vi "_TBD Get Templates Folder Location.vi"() -> (0 "Templates Folder Location":path)   [LabVIEW 2022 SP3]
doc: "Returns the folder location where template VIs and/or CTLs are expected to be found."
panel:
  # "Development\ncontrols/indicators useful for development and testing, but which are not outputs of the VI"
  # "Input\nInputs to the VI"
  # "Output\nOutputs of the VI"
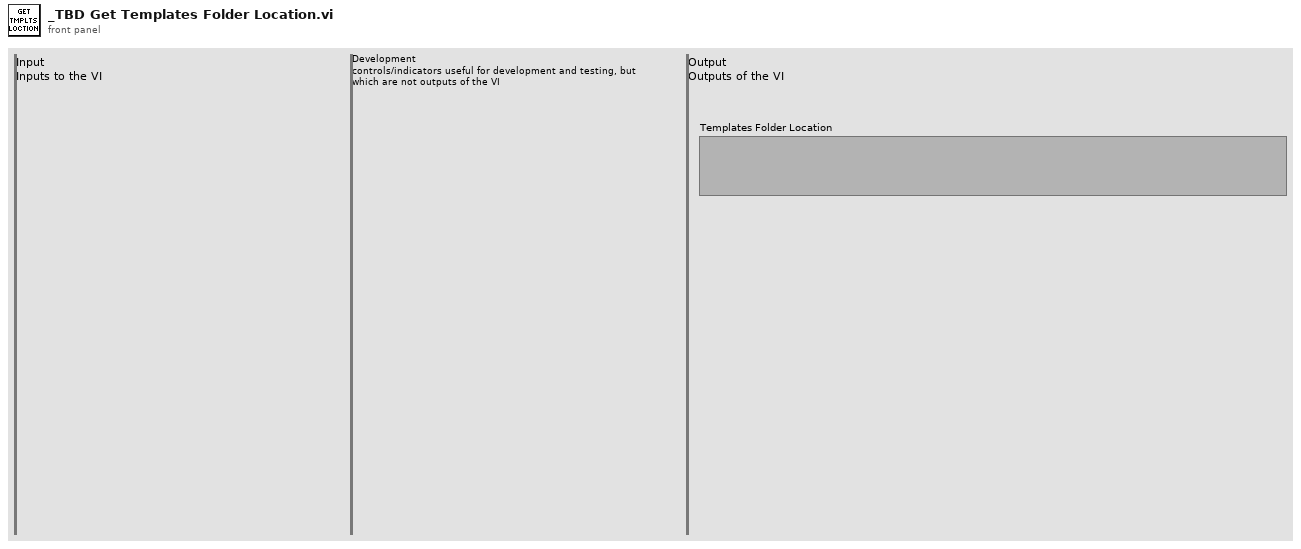
[diagram p1: front panel]
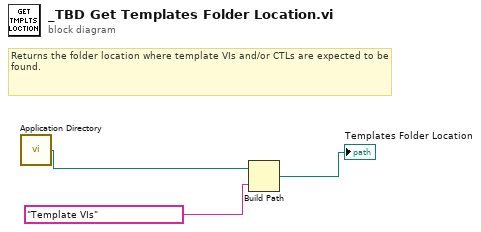
[diagram p0: block diagram]
diagram:
  # "Returns the folder location where template VIs and/or CTLs are expected to be found."
  n1 = call <vilib>:"Application Directory.vi"() -> ("Application Directory"=w1:path)
  n2 = Build Path(base path=w1, name or relative path="Template VIs") -> (appended path=→"Templates Folder Location":path)
